vi "WaitForBlockDone.vi"(8 "error in (no error)":errorcluster) -> (0 "error out":errorcluster)   [LabVIEW 2015, in "ESLSCDLL.lvlib"]
uses:
  ESLSCDLL.lvlib
  Globals.vi
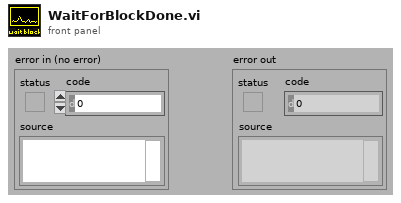
[diagram p1: front panel]
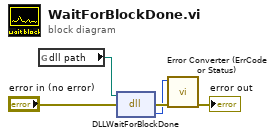
[diagram p0: block diagram]
diagram:
  n1 = global read "Globals.vi" "dll path"() -> (w1:path)
  n2 = dll-call lib="C:/ENTW/PCIE/LV64/board.vis/ESLSCDLL.dll" fn="DLLWaitForBlockDone" ("lwlscdll.dll:DLLWriteLongS0")(path in=w1, error in="error in (no error)") -> (error out=w4:errorcluster, "es_status_codes"=w2:i32)  [unwired: 1 in, 1 out]
  n3 = call "Error Converter (ErrCode or Status).vi"("error in (no error)"=w4, "error code"=w2) -> ("error out"=→"error out":errorcluster)  [unwired: 9 in]
